vi "Main.vi"(0 "Start":bool, 5 "Reset":bool, 7 "Pause":bool, 9 "Resume":bool, 11 "Stop":bool caption="awerwe") -> (4 "hour":i32 format="%0#2_3f", 6 "min":i32 format="%0#2_3f", 8 "sec":i32 format="%0#2_3f", 10 "ms":dbl format="%0#3.0f")   [LabVIEW 2020, in "StopWatch.lvlib"]
doc: "This VI is a simple stop watch."
uses:
  StopWatch.lvlib
  Typedef/Data cluster.ctl
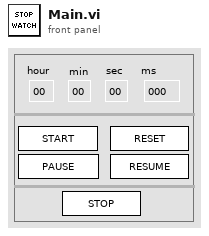
[diagram p1: front panel]
types:
  T1 = typedef "Data cluster.ctl" = cluster{"StartTime":ext, "Timer":ext, "Start":bool, "Pause":bool, "Reset":bool}
  T2 = typedef "LVDateTimeRec.ctl" = cluster{"fractional second":dbl, "second":i32, "minute":i32, "hour":i32, "day of month":i32, "month":i32, "year":i32, "day of week":i32, "day of year":i32, "DST":i32}
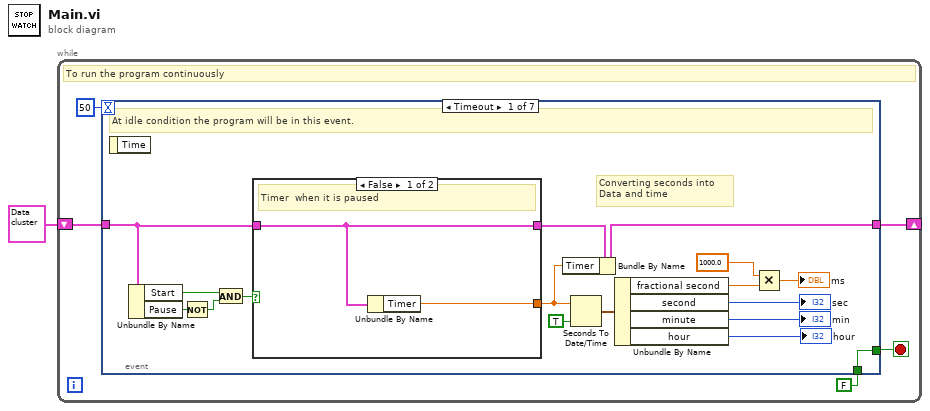
[diagram p0: block diagram]
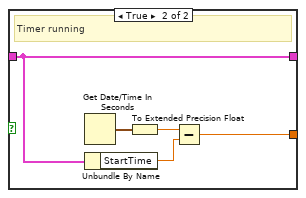
[diagram p2: hidden frame]
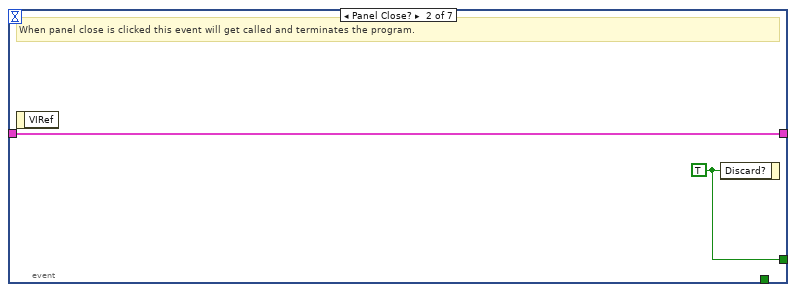
[diagram p3: hidden frame]
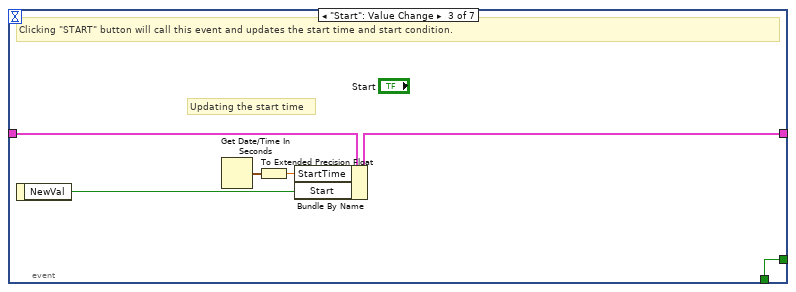
[diagram p4: hidden frame]
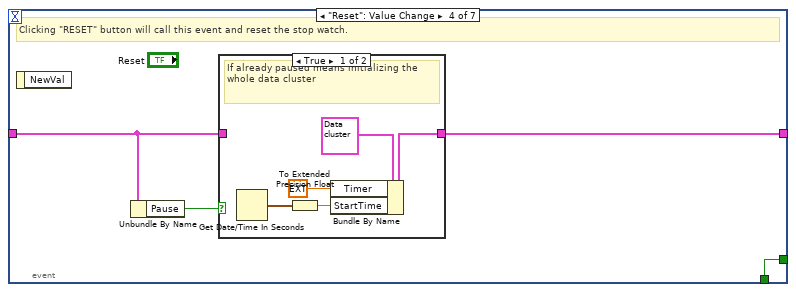
[diagram p5: hidden frame]
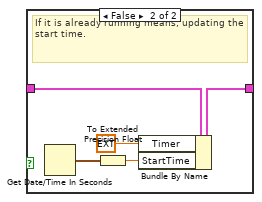
[diagram p6: hidden frame]
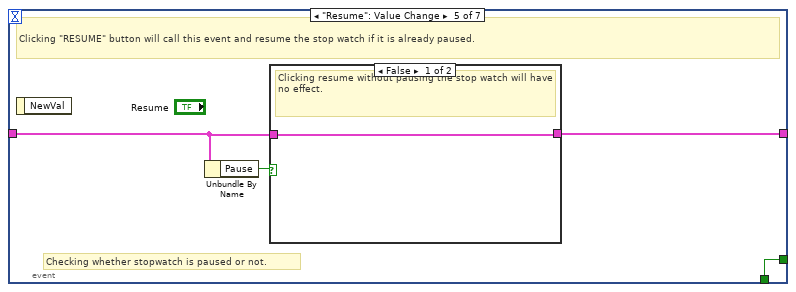
[diagram p7: hidden frame]
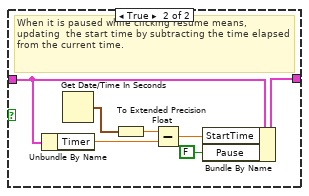
[diagram p8: hidden frame]
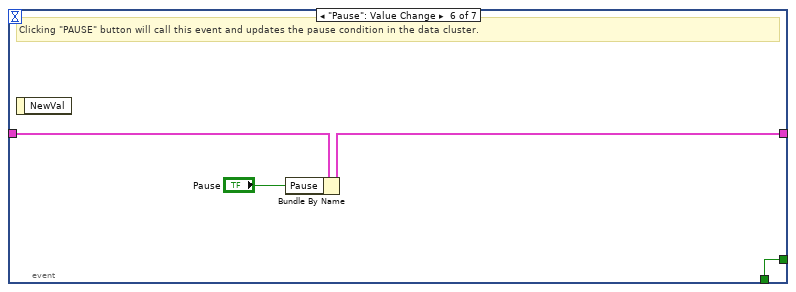
[diagram p9: hidden frame]
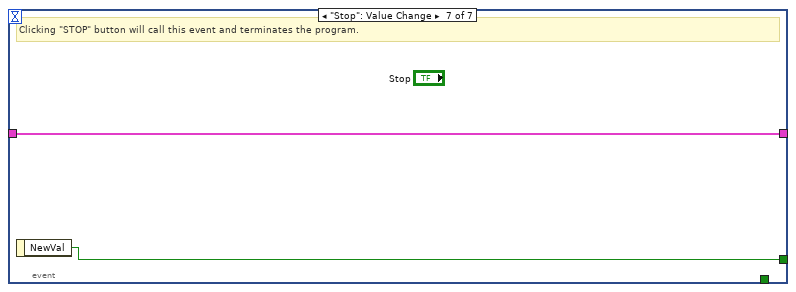
[diagram p10: hidden frame]
diagram:
  n1 = while {
    shift-right: [w5] -> _
    shift-left: T1 {"StartTime"=0.0, "Timer"=0.0, "Start"=FALSE, "Pause"=FALSE, "Reset"=FALSE} -> [w4]
    stop <- w2 stop-if-true
    # "To run the program continuously"
    n2 = event shown="[0] Timeout" {
      selector: _ -> [_ _ _ _ _ _ _]
      dyn-events: _ -> [_ _ _ _ _ _ _]
      timeout: 50 -> [_ _ _ _ _ _ _]
      tunnel: [w7 w31 w33 w39 w53 w65 w69] -> w2
      tunnel: [w12 w32 w36 w42 w56 w68 w70] -> w5
      tunnel: w4 -> [w19 w32 w35 w40 w55 w67 w70]
      tunnel: FALSE ("NewVal") -> [w7 _ w33 w39 w53 w65 _]
      event Timeout {
        # "Converting seconds into\nData and time"
        # "At idle condition the program will be in this event."
        n3 = event-data() -> ()  [unwired: 1 in, 1 out]
        n4 = Unbundle By Name(w19) -> ("Start"=w17:bool, "Pause"=w18:bool)
        n5 = Not(x=w18) -> (.not. x?=w16:bool)
        n6 = And(x=w17, y=w16) -> (x .and. y?=w15:bool)
        n7 = case shown="False" w15 {
          tunnel: [w24 w26] -> w11
          tunnel: [w25 w27] -> w13
          tunnel: w19 -> [w25 w27]
          frame False {
            # "Timer  when it is paused"
            n8 = Unbundle By Name(w25) -> ("Timer"=w24:ext)
          }
          frame True {
            # "Timer running"
            n9 = Get Date/Time In Seconds() -> (seconds since 1Jan1904=w30:timestamp)
            n10 = Unbundle By Name(w27) -> ("StartTime"=w28:ext)
            n11 = To Extended Precision Float(1:w30) -> (0:w29:ext)
            n12 = Subtract(x=w29, y=w28) -> (x-y=w26:ext)
          }
        }
        n13 = Bundle By Name(cluster=w13, "Timer"=w11) -> (w12:T1)
        n14 = Seconds To Date/Time(time stamp (now)=w11, to UTC (F)=TRUE) -> (date time rec=w23:T2)
        n15 = Unbundle By Name(w23) -> ("fractional second"=w10:dbl, "second"=→"sec":i32, "minute"=→"min":i32, "hour"=→"hour":i32)
        n16 = Multiply(x=1000.0 ("y"), y=w10) -> (x*y=→"ms":dbl)
      }
      event Panel Close? {
        w31 = TRUE ("Discard?")
        # "When panel close is clicked this event will get called and terminates the program."
        n17 = event-data() -> ()  [unwired: 1 in, 1 out]
        n18 = event-data("Discard?"=w31) -> ()  [unwired: 1 in, 1 out]
      }
      event "Start": Value Change {
        # "Updating the start time"
        # "Clicking \"START\" button will call this event and updates the start time and start condition."
        n19 = event-data() -> ("NewVal"=w34:bool)  [unwired: 1 in]
        n20 = Get Date/Time In Seconds() -> (seconds since 1Jan1904=w37:timestamp)
        n21 = To Extended Precision Float(1:w37) -> (0:w38:ext)
        n22 = Bundle By Name(cluster=w35, "StartTime"=w38, "Start"=w34) -> (w36:T1)
      }
      event "Reset": Value Change {
        # "Clicking \"RESET\" button will call this event and reset the stop watch."
        n23 = event-data() -> ()  [unwired: 1 in, 1 out]
        n24 = Unbundle By Name(w40) -> ("Pause"=w41:bool)
        n25 = case shown="True" w41 {
          tunnel: [w47 w52] -> w42
          tunnel: w40 -> [_ w48]
          frame True {
            # "If already paused means initializing the whole data cluster"
            n26 = Get Date/Time In Seconds() -> (seconds since 1Jan1904=w45:timestamp)
            n27 = To Extended Precision Float(1:w45) -> (0:w44:ext)
            n28 = Bundle By Name(cluster=T1 {"StartTime"=0.0, "Timer"=0.0, "Start"=FALSE, "Pause"=FALSE, "Reset"=FALSE}, "Timer"=ext 0.0, "StartTime"=w44) -> (w47:T1)
          }
          frame False {
            # "If it is already running means, updating the start time."
            n29 = Get Date/Time In Seconds() -> (seconds since 1Jan1904=w50:timestamp)
            n30 = To Extended Precision Float(1:w50) -> (0:w49:ext)
            n31 = Bundle By Name(cluster=w48, "Timer"=ext 0.0, "StartTime"=w49) -> (w52:T1)
          }
        }
      }
      event "Resume": Value Change {
        # "Checking whether stopwatch is paused or not."
        # "Clicking \"RESUME\" button will call this event and resume the stop watch if it is already paused."
        n32 = event-data() -> ()  [unwired: 1 in, 1 out]
        n33 = Unbundle By Name(w55) -> ("Pause"=w54:bool)
        n34 = case shown="False" w54 {
          tunnel: [w57 w62] -> w56
          tunnel: w55 -> [w57 w61]
          frame False {
            # "Clicking resume without pausing the stop watch will have no effect."
          }
          frame True {
            # "When it is paused while clicking resume means, updating  the start time by subtracting the time elapsed from the current time."
            n35 = Unbundle By Name(w61) -> ("Timer"=w64:ext)
            n36 = Get Date/Time In Seconds() -> (seconds since 1Jan1904=w59:timestamp)
            n37 = To Extended Precision Float(1:w59) -> (0:w58:ext)
            n38 = Subtract(x=w58, y=w64) -> (x-y=w63:ext)
            n39 = Bundle By Name(cluster=w61, "StartTime"=w63, "Pause"=FALSE) -> (w62:T1)
          }
        }
      }
      event "Pause": Value Change {
        # "Clicking \"PAUSE\" button will call this event and updates the pause condition in the data cluster."
        n40 = event-data() -> ()  [unwired: 1 in, 1 out]
        n41 = Bundle By Name(cluster=w67, "Pause"="Pause") -> (w68:T1)
      }
      event "Stop": Value Change {
        # "Clicking \"STOP\" button will call this event and terminates the program."
        n42 = event-data() -> ("NewVal"=w69:bool)  [unwired: 1 in]
      }
    }
  }
